vi "Find Tests - When Project Contains Theory - Returns One Test Case For Each Theory.vi"() -> ()   [LabVIEW 2017, in "LVUnit Test Discoverer.Tests.lvlib"]
uses:
  LVUnit Test Discoverer.Tests.lvlib
  LVUnit Test Discoverer/LVUnit Test Discoverer.lvclass
  <vilib>/PNR/Transparent Assertions/Transparent Assertions/Assertions/Assertions.lvlib
  Test Case/Test Case.lvclass
panel:
  out "error out":errorcluster
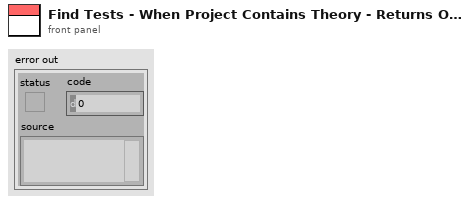
[diagram p1: front panel]
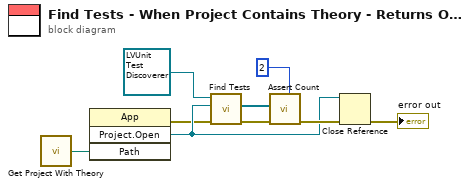
[diagram p0: block diagram]
diagram:
  n1 = call "Get Project With Theory.vi"() -> ("Project File"=w1:path)  [unwired: 2 in]
  n2 = invoke class="App" method="Project.Open"("Path"=w1) -> (error out=w2:errorcluster, "Project:Open"=w3:refnum<vi>)  [unwired: 3 in, 2 out]
  n3 = call-dynamic "Find Tests.vi"("error in (no error)"=w2, "Project Refnum"=w3, "LVUnit Test Discoverer in"=refnum<class "LVUnit Test Discoverer.lvclass"> refnum ("LVUnit Test Discoverer")) -> ("error out"=w8:errorcluster, "Test Cases"=w6:refnum<class "Test Case.lvclass">[])  [unwired: 6 in, 1 out]
  n4 = call <vilib>:"Assert Count.vi"("Expected"=2, "error in (no error)"=w8, "Haystack"=w6) -> ("error out"=w7:errorcluster)  [unwired: 8 in]
  n5 = Close Reference(reference=w3, error in (no error)=w7) -> (error out=→"error out":errorcluster)
